vi "CreateIconClass.vi"(0 "Icon输入":refnum<class "Icon.lvclass">, 1 "settings":T1, 2 "[user-specified font]":T3={"Font Name:"="Arial", "Size"=7, "Strikeout?"=FALSE, "Italic?"=FALSE, "Underline?"=FALSE, "Outline?"=FALSE, "Shadow?"=FALSE, "Bold?"=FALSE}, 5 "lv_icon.lvlib:Icon.lvclass out":refnum<class "Icon.lvclass">, 7 "CommonSettings":T4={"UseLibIcon"=FALSE, "UseIcon"=FALSE, "IconPosition"={"left"=2, "top"=17, "right"=32, "bottom"=32}, "UseText"=FALSE, "TextPosition"={"left"=2, "top"=17, "right"=32, "bottom"=32}}, 9 "CurrentItemSettings":T5, 11 "error in (no error)":errorcluster) -> (4 "Icon输出":refnum<class "Icon.lvclass">, 6 "簇输出":T5, 15 "error out":errorcluster)   [LabVIEW 2015]
uses:
  1_ctl/Item.ctl
  1_ctl/led-new-small.ctl
  <vilib>/LabVIEW Icon API/lv_icon/Classes/Icon/Icon.lvclass
  1_ctl/Settings.ctl
  3_SystemConfiguration/SytleConfigurationDB/Settings-Style/1_Ctl/DB_UUT.ctl
  1_ctl/Ctl-Color.ctl
  <vilib>/LabVIEW Icon API/API_User Layer Data.ctl
  <vilib>/Utility/miscctls.llb/LVPoint32TypeDef.ctl
  <vilib>/picture/picture.llb/imagedata.ctl
  <vilib>/Utility/miscctls.llb/LVBoundsTypeDef.ctl
  <vilib>/LabVIEW Icon API/LabVIEW Icon API.lvlib
  3_SystemConfiguration/SytleConfigurationDB/Settings-Style.lvlib
panel:
  # "Style Settings"
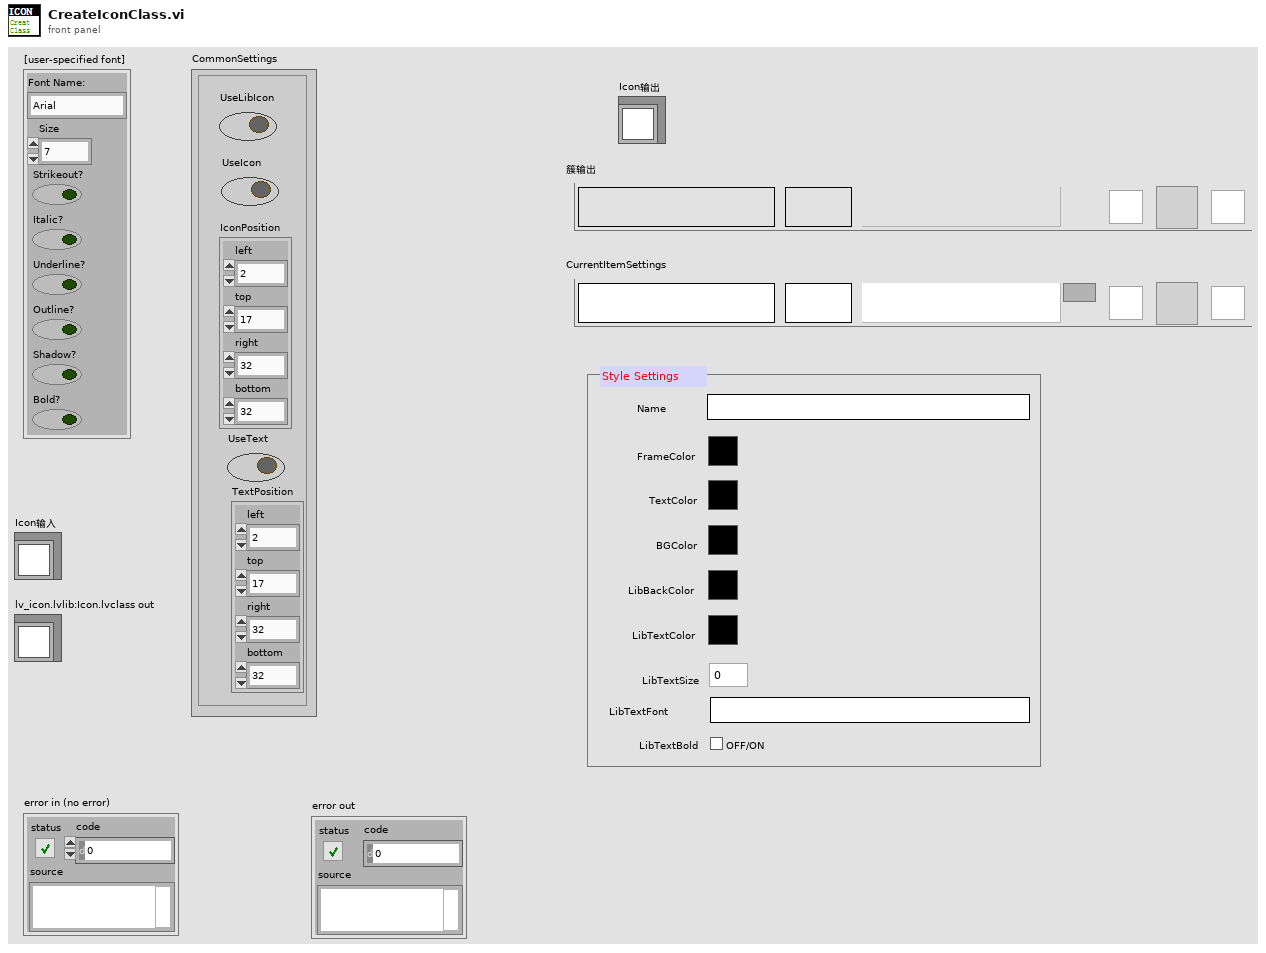
[diagram p1: front panel]
types:
  T1 = typedef "Settings-Style.lvlib/DB_UUT.ctl" = cluster{"Name":string, "FrameColor":T2, "TextColor":T2, "BGColor":T2, "LibBackColor":T2, "LibTextColor":T2, "LibTextSize":u32, "LibTextFont":string, "LibTextBold":bool}
  T2 = typedef "Ctl-Color.ctl" = u32
  T3 = cluster{"Font Name:":string, "Size":i16, "Strikeout?":bool, "Italic?":bool, "Underline?":bool, "Outline?":bool, "Shadow?":bool, "Bold?":bool}
  T4 = typedef "Settings.ctl" = cluster{"UseLibIcon":bool, "UseIcon":bool, "IconPosition":cluster{"left":i16, "top":i16, "right":i16, "bottom":i16}, "UseText":bool, "TextPosition":cluster{"left":i16, "top":i16, "right":i16, "bottom":i16}}
  T5 = typedef "Item.ctl" = cluster{"New Icon":picture, "Vi Name":string, "Old Icon":picture, "Text":string, "SpecialIcon":path, "Update":T6, "path":path}
  T6 = typedef "led-new-small.ctl" = bool
  T7 = typedef "LabVIEW Icon API.lvlib/API_User Layer Data.ctl" = cluster{"Layer name":string, "Origin":T8, "Icon image data":T9}
  T8 = typedef "LVPoint32TypeDef.ctl" = cluster{"Horizontal":i32, "Vertical":i32}
  T9 = typedef "imagedata.ctl" = cluster{"image type":i32, "image depth":i32, "image":u8[], "mask":u8[], "colors":u32[], "Rectangle":cluster{"left":i16, "top":i16, "right":i16, "bottom":i16}}
  T10 = cluster{"left":i16, "top":i16, "right":i16, "bottom":i16}
  T11 = typedef "LVBoundsTypeDef.ctl" = cluster{"Width":u32, "Height":u32}
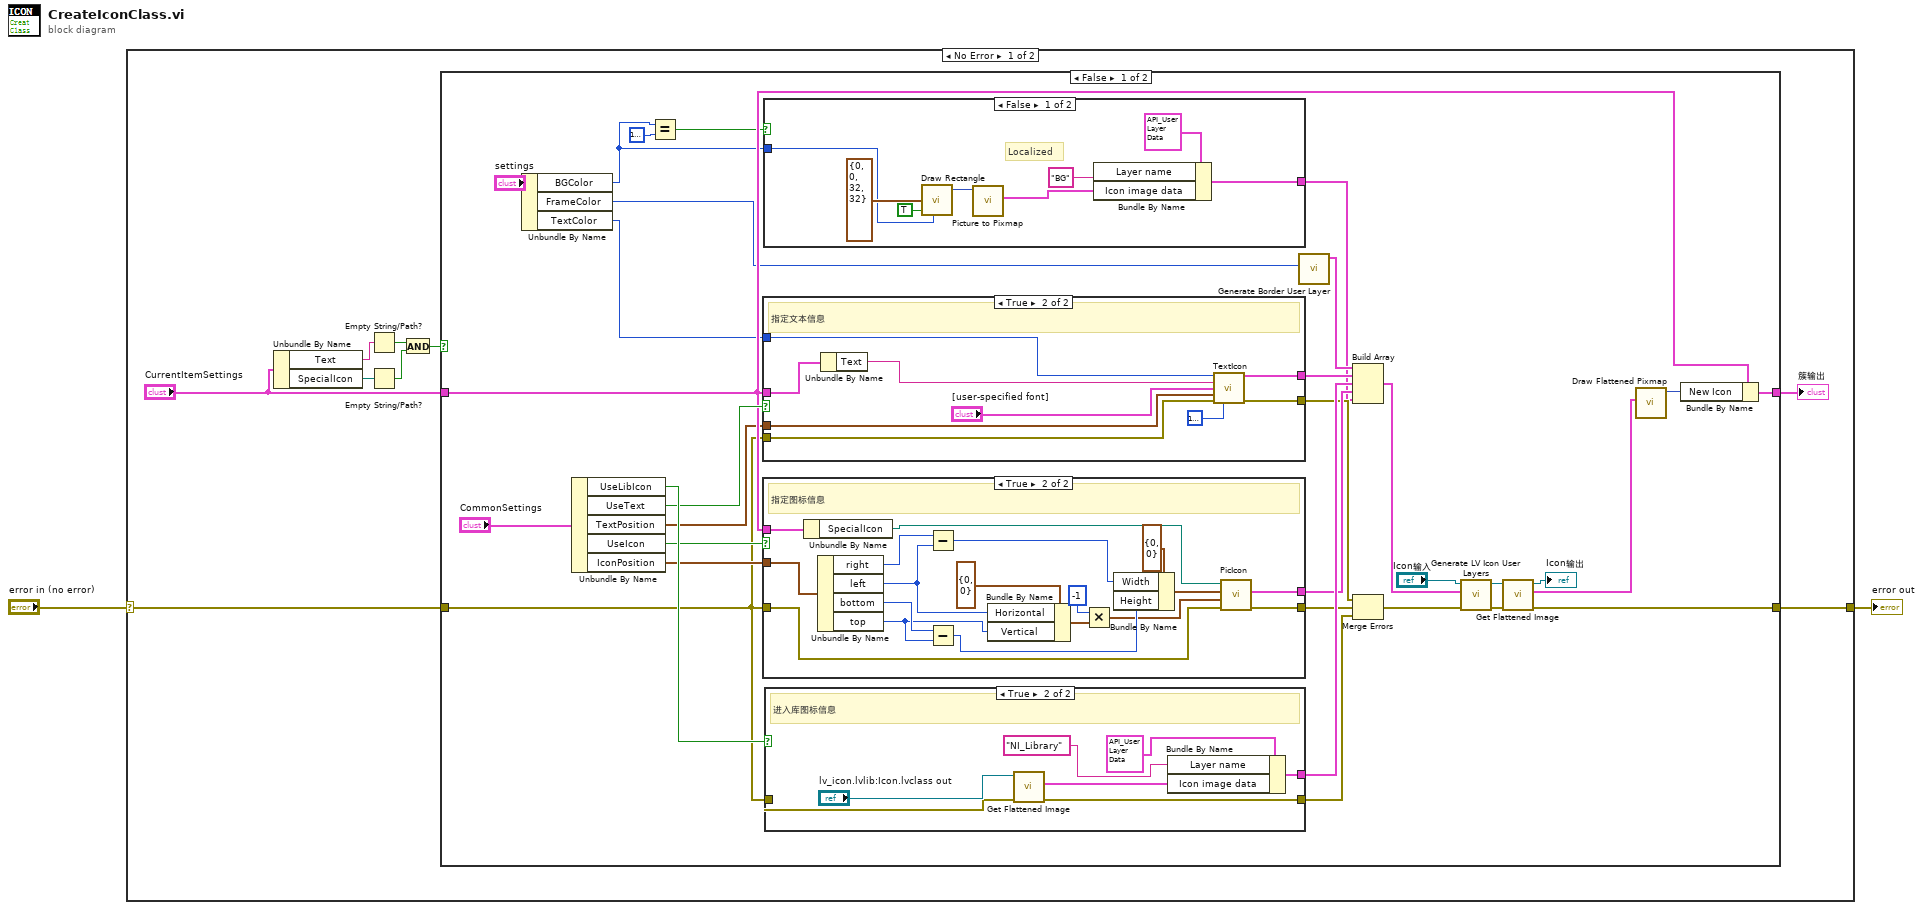
[diagram p0: block diagram]
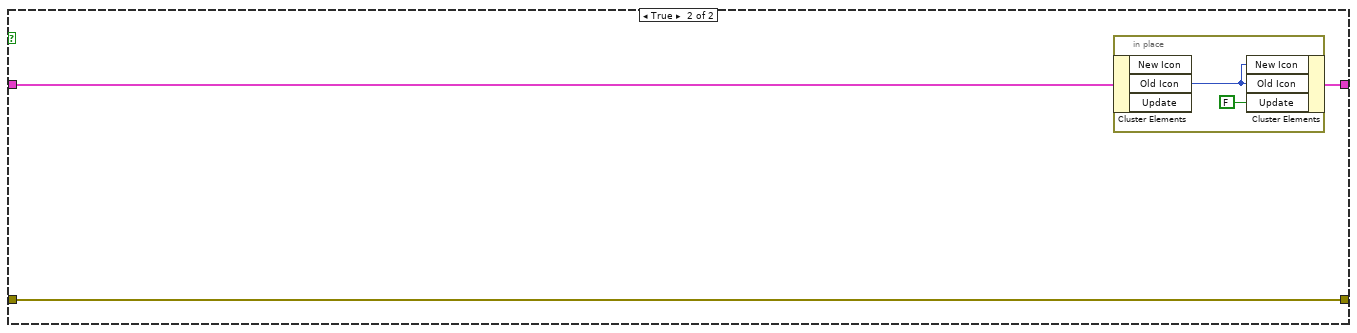
[diagram p6: hidden frame]
diagram:
  n1 = case shown="No Error" "error in (no error)" {
    selector: "error in (no error)" -> [w4 w94]
    tunnel: [w3 w94] -> w1
    frame No Error {
      n2 = Unbundle By Name("CurrentItemSettings") -> ("Text"=w10:string, "SpecialIcon"=w9:path)
      n3 = Empty String/Path?(string/path=w10) -> (empty?=w8:bool)
      n4 = Empty String/Path?(string/path=w9) -> (empty?=w7:bool)
      n5 = And(x=w8, y=w7) -> (x .and. y?=w6:bool)
      n6 = case shown="False" w6 {
        tunnel: [w42 w90] -> w11
        tunnel: "CurrentItemSettings" -> [w33 w91]
        tunnel: w4 -> [w26 w89]
        tunnel: [w19 w89] -> w3
        frame False {
          n7 = Unbundle By Name("settings") -> ("BGColor"=w14:T2, "FrameColor"=w13:T2, "TextColor"=w12:T2)
          n8 = Unbundle By Name("CommonSettings") -> ("UseLibIcon"=w36:bool, "UseText"=w35:bool, "TextPosition"=w32:T10, "UseIcon"=w34:bool, "IconPosition"=w31:T10)
          n9 = Equal?(x=w14, y=u32 16777216 ("BG color(transparent)")) -> (x = y?=w17:bool)
          n10 = case shown="True" w35 {
            tunnel: w33 -> [_ w79]
            tunnel: w32 -> [_ w78]
            tunnel: w26 -> [w71 w76]
            tunnel: [w71 w75] -> w24
            tunnel: [_ w74] -> w29
            tunnel: w12 -> [_ w72]
            frame False {
            }
            frame True {
              # "指定文本信息"
              n11 = Unbundle By Name(w79) -> ("Text"=w80:string)
              n12 = call "TextIcon.vi"(0:"Text"=w72, 5:"Text"=w80, "[user-specified font]"="[user-specified font]", "rect"=w78, "error in (no error)"=w76, "BG color(transparent)"=u32 16777216) -> (">> TextIcon >>"=w74:T7, "error out"=w75:errorcluster)  [unwired: 8 in]
            }
          }
          n13 = case shown="True" w34 {
            tunnel: w33 -> [_ w70]
            tunnel: w31 -> [_ w66]
            tunnel: w26 -> [w52 w57]
            tunnel: [w52 w56] -> w20
            tunnel: [_ w55] -> w27
            frame False {
            }
            frame True {
              # "指定图标信息"
              n14 = Unbundle By Name(w70) -> ("SpecialIcon"=w69:path)
              n15 = Unbundle By Name(w66) -> ("right"=w65:i16, "left"=w59:i16, "bottom"=w64:i16, "top"=w58:i16)
              n16 = Subtract(x=w65, y=w59) -> (x-y=w63:i16)
              n17 = Subtract(x=w64, y=w58) -> (x-y=w62:i16)
              n18 = Bundle By Name(cluster=T8 {"Horizontal"=0, "Vertical"=0} ("Origin"), "Horizontal"=w59, "Vertical"=w58) -> (w60:T8)
              n19 = Multiply(x=-1, y=w60) -> (x*y=w54:T8)
              n20 = Bundle By Name(cluster=T11 {"Width"=0, "Height"=0} ("Size"), "Width"=w63, "Height"=w62) -> (w67:T11)
              n21 = call "PicIcon.vi"("error in (no error)"=w57, "Origin"=w54, "Size"=w67, "FilePath"=w69) -> ("error out"=w56:errorcluster, "IconClass"=w55:T7)  [unwired: 6 in]
            }
          }
          n22 = case shown="False" w17 {
            tunnel: [w46 _] -> w16
            tunnel: w14 -> [w44 _]
            frame False {
              # "Localized"
              n23 = call <vilib>:"Draw Rectangle.vi"("rect"=T10 {"left"=0, "top"=0, "right"=32, "bottom"=32}, "fill?(F)"=TRUE, "color(black)"=w44) -> ("new picture"=w50:picture)  [unwired: 6 in]
              n24 = call <vilib>:"Picture to Pixmap.vi"("picture"=w50) -> ("image data"=w51:T9)  [unwired: 9 in, 1 out]
              n25 = Bundle By Name(cluster=T7 {"Layer name"="", "Origin"={"Horizontal"=0, "Vertical"=0}, "Icon image data"={"image type"=0, "image depth"=0, "image"=[], "mask"=[], "colors"=[], "Rectangle"={"left"=0, "top"=0, "right"=0, "bottom"=0}}} ("User layer"), "Layer name"="BG" ("Border"), "Icon image data"=w51) -> (w46:T7)
            }
            frame True {
            }
          }
          n26 = case shown="True" w36 {
            tunnel: w26 -> [w81 w84]
            tunnel: [w81 w83] -> w23
            tunnel: [_ w82] -> w28
            frame False {
            }
            frame True {
              # "进入库图标信息"
              n27 = call <vilib>:"Get Flattened Image.vi"("error in (no error)"=w84, "lv_icon.lvlib:Icon.lvclass in"="lv_icon.lvlib:Icon.lvclass out") -> ("error out"=w83:errorcluster, "Color Image"=w87:T9)  [unwired: 6 in, 2 out]
              n28 = Bundle By Name(cluster=T7 {"Layer name"="", "Origin"={"Horizontal"=0, "Vertical"=0}, "Icon image data"={"image type"=0, "image depth"=0, "image"=[], "mask"=[], "colors"=[], "Rectangle"={"left"=0, "top"=0, "right"=0, "bottom"=0}}} ("User layer"), "Layer name"="NI_Library", "Icon image data"=w87) -> (w82:T7)
            }
          }
          n29 = call <vilib>:"Generate Border User Layer.vi"("color(black)"=w13) -> ("User Layer data"=w30:T7)  [unwired: 10 in]
          n30 = Build Array(w30, w29, w28, w27, w16) -> (w25:T7[])
          n31 = Merge Errors(w24, w20, w23) -> (w22:errorcluster)
          n32 = call <vilib>:"Generate LV Icon User Layers.vi"("error in (no error)"=w22, "User layers"=w25, "Icon in"="Icon输入") -> ("error out"=w21:errorcluster, "Icon out"=w38:refnum<class "Icon.lvclass">)  [unwired: 7 in]
          n33 = call <vilib>:"Get Flattened Image.vi"("error in (no error)"=w21, "lv_icon.lvlib:Icon.lvclass in"=w38) -> ("error out"=w19:errorcluster, "Color Image"=w40:T9, "lv_icon.lvlib:Icon.lvclass out"=→"Icon输出":refnum<class "Icon.lvclass">)  [unwired: 6 in, 1 out]
          n34 = call <vilib>:"Draw Flattened Pixmap.vi"("image data"=w40) -> ("new picture"=w39:picture)  [unwired: 8 in]
          n35 = Bundle By Name(cluster=w33, "New Icon"=w39) -> (w42:T5)
        }
        frame True {
          n36 = in-place {
            n37 = in-place-cluster #1(w91) -> ("Old Icon"=w93:picture)  [unwired: 2 out]
            n38 = in-place-cluster #1("New Icon"=w93, "Old Icon"=w93, "Update"=FALSE) -> (w90:T5)
          }
        }
      }
      "簇输出" <- w11
    }
    frame Error {
    }
  }
  "error out" <- w1
